vi "Read Current Position.vi"(8 "error in (no error)":errorcluster, 11 "Double Scanner.lvclass":refnum<class "Double Scanner.lvclass">) -> (0 "error out":errorcluster, 1 "Pos 2":dbl, 2 "Pos 1":dbl, 3 "Double Scanner.lvclass 2":refnum<class "Double Scanner.lvclass">)   [LabVIEW 2012, in "Double Scanner.lvclass"]
uses:
  Double Scanner.lvclass
  Scanner/Scanner.lvclass
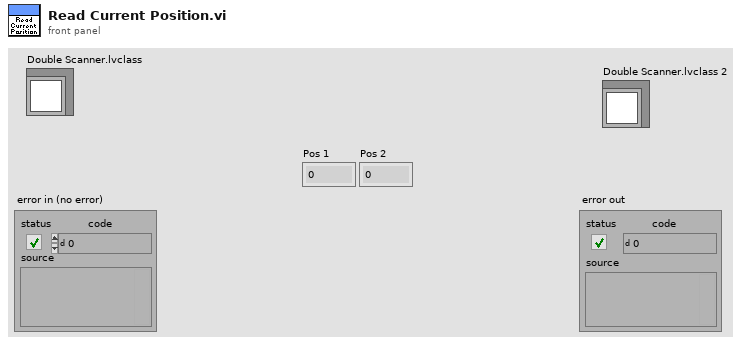
[diagram p1: front panel]
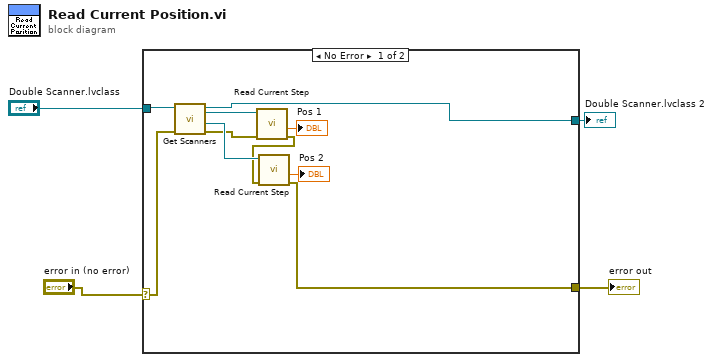
[diagram p0: block diagram]
diagram:
  n1 = case shown="No Error" "error in (no error)" {
    selector: "error in (no error)" -> [w8 w16]
    tunnel: [w5 w16] -> w3
    tunnel: "Double Scanner.lvclass" -> [w14 w15]
    tunnel: [w9 w15] -> w1
    frame No Error {
      n2 = call-dynamic "Get Scanners.vi"("error in (no error)"=w8, "Double Scanner in"=w14) -> ("error out"=w7:errorcluster, "Scanner 2 out"=w12:refnum<class "Scanner.lvclass">, "Scanner 1 out"=w13:refnum<class "Scanner.lvclass">, "Double Scanner out"=w9:refnum<class "Double Scanner.lvclass">)  [unwired: 6 in]
      n3 = call-dynamic "Read Current Step.vi"("error in (no error)"=w7, "Scanner.lvclass in"=w13) -> ("error out"=w6:errorcluster, "Current Position"=→"Pos 1":dbl)  [unwired: 6 in, 2 out]
      n4 = call-dynamic "Read Current Step.vi"("error in (no error)"=w6, "Scanner.lvclass in"=w12) -> ("error out"=w5:errorcluster, "Current Position"=→"Pos 2":dbl)  [unwired: 6 in, 2 out]
    }
    frame Error {
    }
  }
  "Double Scanner.lvclass 2" <- w1
  "error out" <- w3
